vi "drop_thresh.vi"(10 "threshold":dbl format="%#_13g", 11 "curve":dbl[](array[numeric])) -> (3 "position":dbl)   [LabVIEW 2016]
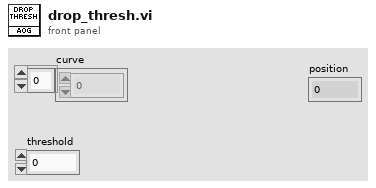
[diagram p1: front panel]
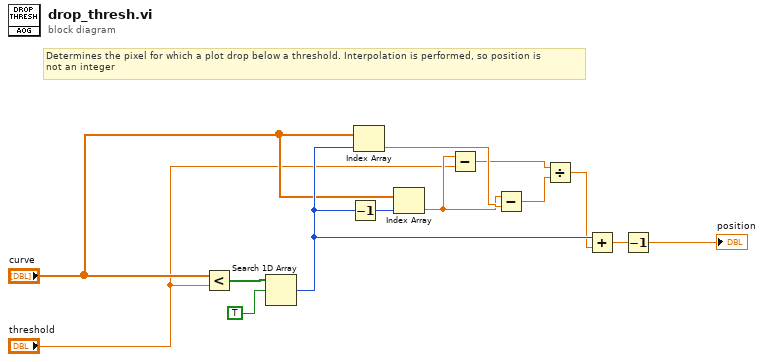
[diagram p0: block diagram]
diagram:
  # "Determines the pixel for which a plot drop below a threshold. Interpolation is performed, so position is\nnot an integer"
  n1 = Less?(x="curve", y="threshold") -> (x < y?=w13:bool[])
  n2 = Search 1D Array(1D array=w13, element=TRUE) -> (index of element=w10:i32)  [unwired: 1 in]
  n3 = Decrement(x=w10) -> (x-1=w11:i32)
  n4 = Index Array(array="curve", index=w10) -> (element=w8:dbl)
  n5 = Index Array(array="curve", index=w11) -> (element=w7:dbl)
  n6 = Subtract(x=w7, y="threshold") -> (x-y=w6:dbl)
  n7 = Subtract(x=w7, y=w8) -> (x-y=w5:dbl)
  n8 = Divide(x=w6, y=w5) -> (x/y=w9:dbl)
  n9 = Add(x=w10, y=w9) -> (x+y=w4:dbl)
  n10 = Decrement(x=w4) -> (x-1=→"position":dbl)
